vi "SavePowerLimits.vi"(8 "error in (no error)":errorcluster caption="Fehler (Eingang, kein Fehler)", 11 "device":u32) -> (0 "error out":errorcluster caption="Fehler (Ausgang)", 3 "function return":u32(ring))   [LabVIEW 2015, in "IRB.lvlib"]
doc: "irb_result IRB_EXPORT irb_save_power_limits(irb_device* device);"
uses:
  IRB.lvlib
  IRB.dll
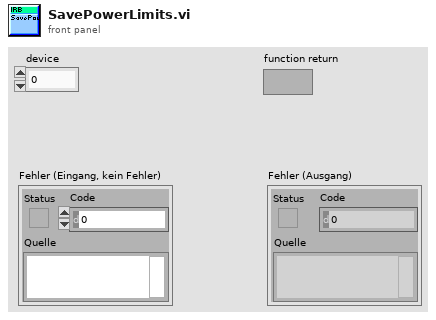
[diagram p1: front panel]
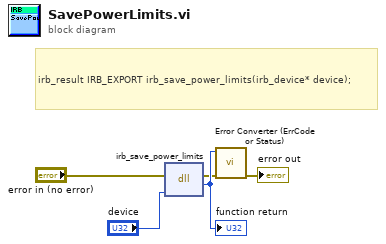
[diagram p0: block diagram]
diagram:
  # "irb_result IRB_EXPORT irb_save_power_limits(irb_device* device);"
  n1 = dll-call lib="C:/LabView/IRB/x86_32/IRB.*" fn="irb_save_power_limits"(error in="error in (no error)", "device"="device") -> (error out=w2:errorcluster, w5:u32)  [unwired: 3 in, 1 out]
  "function return" <- w5
  n2 = call "Error Converter (ErrCode or Status).vi"("error in (no error)"=w2, "error code"=w5) -> ("error out"=→"error out":errorcluster)  [unwired: 9 in]
